vi "FTW-Actor-GetNextJob.vi"(8 "error in":errorcluster, 10 "Jobs Performed":i32, 11 "FTW Actor Instance":refnum<class "FTW-ActorInstance.lvclass">) -> (0 "error out":errorcluster, 1 "Job Data":string, 2 "Job Name":string, 3 "FTW Actor Instance out":refnum<class "FTW-ActorInstance.lvclass">)   [LabVIEW 2013, in "FTW-ActorInstance.lvclass"]
uses:
  FTW-ActorInstance.lvclass
  FTW-ActorInstance.lvclass/FTW-ActorInstance.ctl
  JobSequencer/FTW-JobSequencer.lvclass
panel:
  # "Inputs"
  # "Outputs"
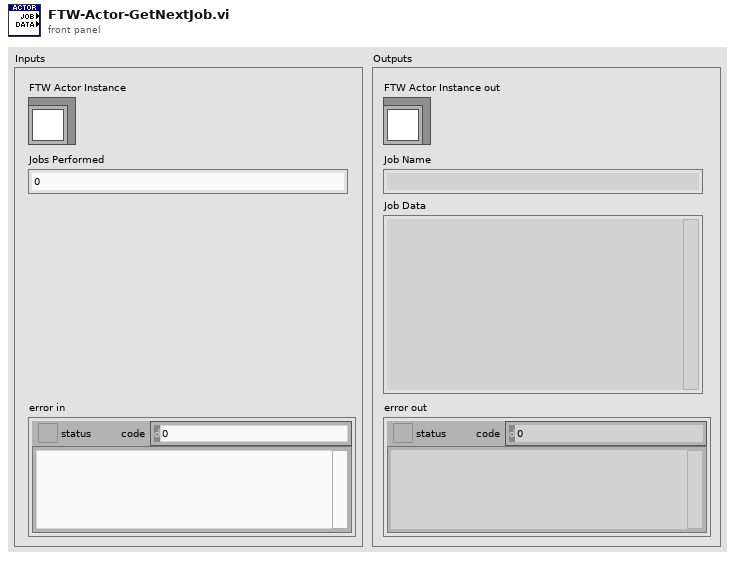
[diagram p1: front panel]
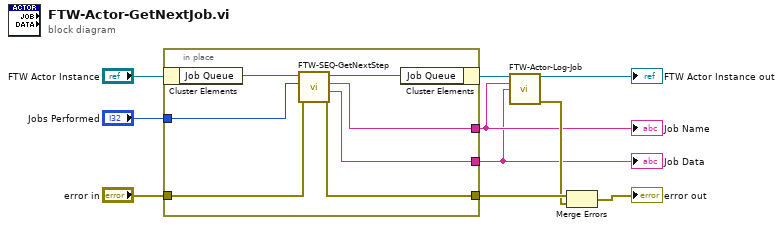
[diagram p0: block diagram]
diagram:
  n1 = in-place {
    in-place-border: "error in" -> [w17]
    in-place-border: [w16] -> w9
    in-place-border: [w13] -> w2
    in-place-border: [w12] -> w1
    in-place-border: "Jobs Performed" -> [w11]
    n2 = in-place-cluster #1("FTW Actor Instance") -> ("Job Queue"=w15:refnum<class "FTW-JobSequencer.lvclass">)
    n3 = call "FTW-SEQ-GetNextStep.vi"("error in"=w17, "Jobs Performed"=w11, "FTW Job Sequencer"=w15) -> ("error out"=w16:errorcluster, "Job Data"=w12:string, "Current Job"=w13:string, "FTW Job Sequencer out"=w14:refnum<class "FTW-JobSequencer.lvclass">)  [unwired: 5 in]
    n4 = in-place-cluster #1("Job Queue"=w14) -> (w8:refnum<class "FTW-ActorInstance.lvclass">)
  }
  "Job Name" <- w2
  "Job Data" <- w1
  n5 = call "FTW-Actor-Log-Job.vi"("FTW Actor Instance"=w8, "Job Name"=w2, "Job Data"=w1) -> ("FTW Actor Instance out"=→"FTW Actor Instance out":refnum<class "FTW-ActorInstance.lvclass">, "error out"=w3:errorcluster)  [unwired: 11 in]
  n6 = Merge Errors(w9, w3) -> (→"error out":errorcluster)
